vi "processCommandSubscribe.vi"(8 "error in (no error)":errorcluster, 11 "MiddlewareSALThisComponent in":refnum<class "MiddlewareSALThisComponent.lvclass">) -> (0 "error out":errorcluster, 3 "MiddlewareSALThisComponent out":refnum<class "MiddlewareSALThisComponent.lvclass">)   [LabVIEW 2016, in "MiddlewareSALThisComponent.lvclass"]
uses:
  MiddlewareSALThisComponent.lvclass
  home/andres/ct_cmpuserevents/ComponentTemplateCore/ComponentModel/ComponentModel/Middleware/Middleware.lvclass
  ComponentTemplateCore/ComponentModel/ComponentModel/Middleware/Middleware.lvclass/Middleware.ctl
  ComponentTemplateCore/ComponentModel/ComponentModel/MiddlewareProcessEvent/MiddlewareProcessEvent.lvclass/MiddlewareProcessEvent.ctl
  ComponentTemplateCore/ComponentModel/ComponentModel/CommandEvent/CommandEvent.lvclass/CommandEvent.ctl
  ProgrammaticInitialization/ProgrammaticInitialization.lvclass
  ComponentTemplateCore/ComponentModel/ComponentModel/Middleware/Middleware.lvclass
  ComponentTemplateCore/ComponentModel/ComponentModel/MiddlewareProcessEvent/MiddlewareProcessEvent.lvclass
  ComponentTemplateCore/ComponentModel/ComponentModel/CommandEvent/CommandEvent.lvclass
panel:
  out "stopIsTrue":bool
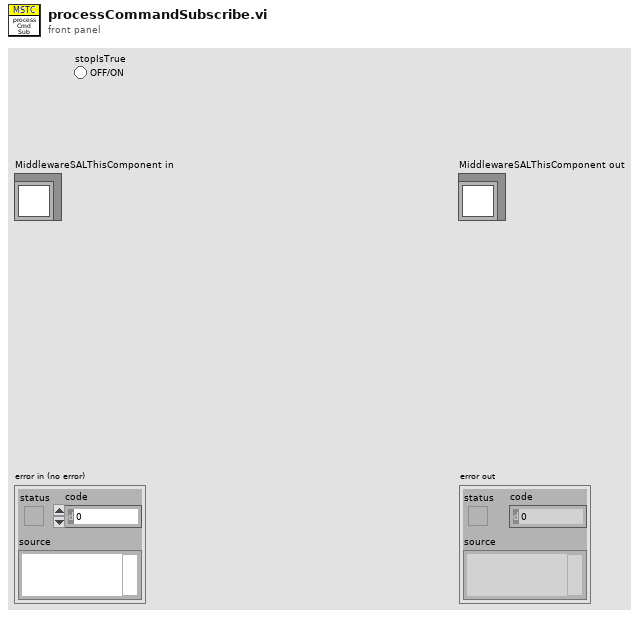
[diagram p1: front panel]
types:
  T1 = typedef "MiddlewareProcessEvents.ctl" = cluster{"disconnect":refnum<user-event>, "error":refnum<user-event>}
  T2 = cluster{"SAL Event Reg Refnum":refnum<event-registration>, "Event Registration Refnum":refnum<event-registration>}
  T3 = typedef "CommandEvents.ctl" = cluster{"command":refnum<user-event>}
  T4 = typedef "SALLV_EXA.lvlib/logevent_InternalCommand.ctl" = cluster{"CommandObject[1000]":u8[], "priority":i32}
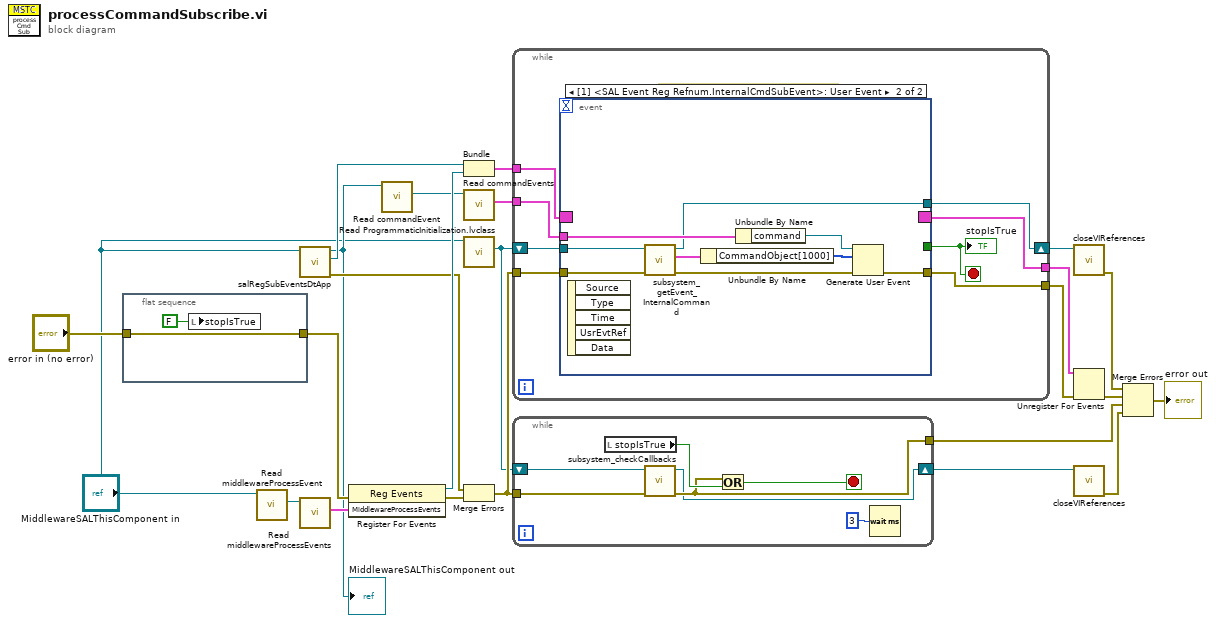
[diagram p0: block diagram]
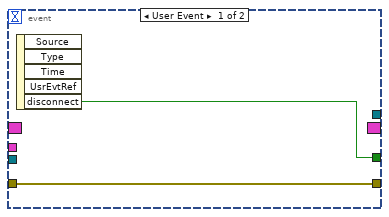
[diagram p2: hidden frame]
diagram:
  n1 = flat-sequence {
    tunnel: "error in (no error)" -> [w26]
    tunnel: [w26] -> w18
    frame #0 {
      n2 = local write "stopIsTrue"(FALSE ("stopIsTrue")) -> ()
    }
  }
  n3 = call "Read middlewareProcessEvent.vi"("Middleware in"="MiddlewareSALThisComponent in") -> ("middlewareProcessEvent"=w24:refnum<class "MiddlewareProcessEvent.lvclass">)  [unwired: 9 in, 1 out]
  n4 = call "salRegSubEventsDtApp.vi"("MiddlewareSALThisComponent in"="MiddlewareSALThisComponent in") -> ("error out"=w14:errorcluster, "SAL Event Reg Refnum"=w16:refnum<event-registration>, "MiddlewareSALThisComponent out"=w13:refnum<class "MiddlewareSALThisComponent.lvclass">)  [unwired: 8 in]
  "MiddlewareSALThisComponent out" <- w13
  n5 = call "Read middlewareProcessEvents.vi"("MiddlewareProcessEvent in"=w24) -> ("MiddlewareProcessEvents"=w23:T1)  [unwired: 9 in, 1 out]
  n6 = register-events(error in=w18, w23) -> (reference out=w21:refnum<event-registration>, error out=w15:errorcluster)  [unwired: 1 in]
  n7 = call "Read commandEvent.vi"("Middleware in"=w13) -> ("commandEvent"=w12:refnum<class "CommandEvent.lvclass">)  [unwired: 9 in, 1 out]
  n8 = Bundle("SAL Event Reg Refnum"=w16, "Event Registration Refnum"=w21) -> (w22:T2)  [unwired: 1 in]
  n9 = call "Read commandEvents.vi"("CommandEvent in"=w12) -> ("CommandEvents"=w11:T3)  [unwired: 9 in, 1 out]
  n10 = call-dynamic "Read ProgrammaticInitialization.lvclass.vi"("MiddlewareSALThisComponent in"="MiddlewareSALThisComponent in") -> ("ProgrammaticInitialization.lvclass"=w5:refnum<class "ProgrammaticInitialization.lvclass">)  [unwired: 8 in, 2 out]
  n11 = Merge Errors(w14, w15) -> (w7:errorcluster)
  n12 = while {
    tunnel: w22 -> [w34]
    tunnel: [w33] -> w20
    tunnel: w7 -> [w31]
    tunnel: [w30] -> w19
    tunnel: w11 -> [w29]
    shift-right: [w27] -> w4
    shift-left: w5 -> [w28]
    stop <- w32 stop-if-true
    # "Check what to do with the error event"
    n13 = event shown="[1] <SAL Event Reg Refnum.InternalCmdSubEvent>: User Event" {
      selector: w34 -> [_ _]
      dyn-events: [_ _] -> w33
      timeout: _ -> [_ _]
      tunnel: [w35 _] -> w32
      tunnel: w31 -> [w36 w40]
      tunnel: [w36 w45] -> w30
      tunnel: w29 -> [_ w44]
      tunnel: w28 -> [_ w38]
      tunnel: [_ w37] -> w27
      event User Event {
        n14 = event-data() -> ("disconnect"=w35:bool)  [unwired: 1 in, 4 out]
      }
      event User Event {
        n15 = event-data() -> ()  [unwired: 1 in, 5 out]
        n16 = call "subsystem_getEvent_InternalCommand.vi"("error in (no error)"=w40, "ProgrammaticInitialization in"=w38) -> ("error out"=w41:errorcluster, "logevent_InternalCommand"=w39:T4, "ProgrammaticInitialization out"=w37:refnum<class "ProgrammaticInitialization.lvclass">)  [unwired: 7 in]
        n17 = Unbundle By Name(w39) -> ("CommandObject[1000]"=w42:u8[])
        n18 = Unbundle By Name(w44) -> ("command"=w43:refnum<user-event>)
        n19 = Generate User Event(user event=w43, event data cluster=w42, error in=w41) -> (error out=w45:errorcluster)  [unwired: 1 in, 1 out]
      }
    }
    "stopIsTrue" <- w32
  }
  n20 = while {
    tunnel: [w49] -> w8
    tunnel: w7 -> [w48]
    shift-right: [w46] -> w2
    shift-left: w5 -> [w47]
    stop <- w50 stop-if-true
    n21 = local read "stopIsTrue"() -> (w51:bool)
    n22 = call "subsystem_checkCallbacks.vi"("error in (no error)"=w48, "ProgrammaticInitialization in"=w47) -> ("error out"=w49:errorcluster, "ProgrammaticInitialization out"=w46:refnum<class "ProgrammaticInitialization.lvclass">)  [unwired: 8 in]
    n23 = Or(x=w49, y=w51) -> (x .or. y?=w50:bool)
    n24 = Wait (ms)(milliseconds to wait=u32 3) -> ()  [unwired: 1 out]
  }
  n25 = call "closeVIReferences.vi"("ProgrammaticInitialization in"=w4) -> ("error out"=w3:errorcluster)  [unwired: 9 in, 1 out]
  n26 = Unregister For Events(event registration refnum=w20, error in=w19) -> (error out=w9:errorcluster)
  n27 = call "closeVIReferences.vi"("ProgrammaticInitialization in"=w2) -> ("error out"=w1:errorcluster)  [unwired: 9 in, 1 out]
  n28 = Merge Errors(w3, w9, w8, w1) -> (→"error out":errorcluster)
